vi "add_Control_panel.vi"(8 "error in (no error)":errorcluster, 10 "VI Refnum out":refnum<vi>, 11 "Control_Ref":refnum<vi>) -> (0 "error out":errorcluster, 3 "New Control Ref":refnum<vi>)   [LabVIEW 2015]
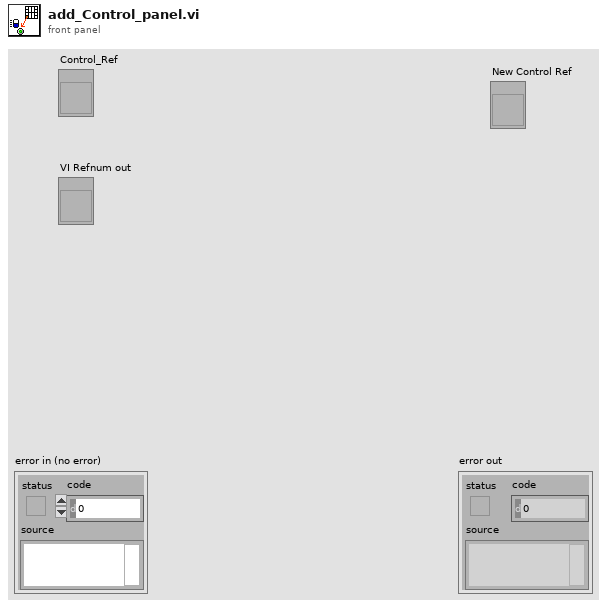
[diagram p1: front panel]
types:
  T1 = enum16{"Invalid Wire Rule", "Required", "Recommended", "Optional", "Dynamic Dispatch"}
  T2 = typedef "LVRectTypeDef.ctl" = cluster{"Left":i16, "Top":i16, "Right":i16, "Bottom":i16}
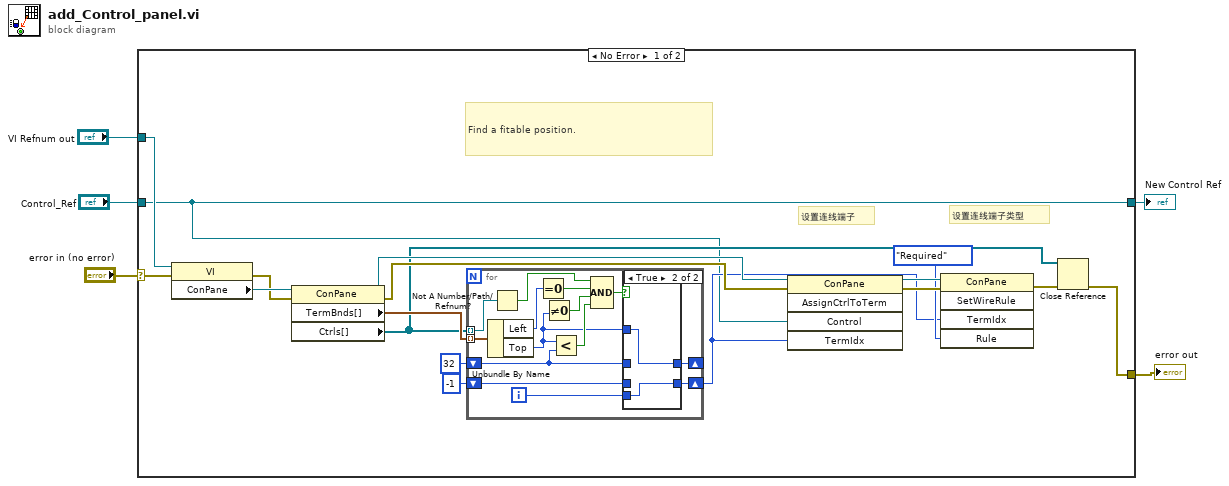
[diagram p0: block diagram]
diagram:
  n1 = case shown="No Error" "error in (no error)" {
    selector: "error in (no error)" -> [w8 w42]
    tunnel: [w7 w42] -> w4
    tunnel: "Control_Ref" -> [w6 w41]
    tunnel: "VI Refnum out" -> [w9 _]
    tunnel: [w6 w41] -> w1
    frame No Error {
      # "设置连线端子"
      # "设置连线端子类型"
      # "Find a fitable position."
      n2 = property class="VI"(reference=w9, error in=w8) -> (error out=w18:errorcluster, "ConPane"=w19:refnum<vi>)  [unwired: 1 out]
      n3 = property class="ConPane"(reference=w19, error in=w18) -> (reference out=w13:refnum<vi>, error out=w14:errorcluster, "TermBnds[]"=w15:T2[], "Ctrls[]"=w10:refnum<vi>[])
      n4 = for {
        tunnel: w15 -> [w26] mode=indexing
        shift-right: [w27] -> _
        shift-left: i16 32 -> [w31]
        shift-right: [w29] -> w12
        shift-left: -1 -> [w30]
        tunnel: w10 -> [w24] mode=indexing
        i -> [w28]
        n5 = Unbundle By Name(w26) -> ("Left"=w25:i16, "Top"=w32:i16)
        n6 = Not A Number/Path/Refnum?(number/path/refnum=w24) -> (NaN/Path/Refnum?=w23:bool)
        n7 = Equal To 0?(x=w25) -> (x = 0?=w36:bool)
        n8 = Not Equal To 0?(x=w32) -> (x != 0?=w35:bool)
        n9 = Less?(x=w32, y=w31) -> (x < y?=w34:bool)
        n10 = Compound Arithmetic op=AND(w23, w36, w35, w34) -> (w33:bool)
        n11 = case shown="True" w33 {
          tunnel: w32 -> [_ w39]
          tunnel: w31 -> [w38 _]
          tunnel: w30 -> [w37 _]
          tunnel: [w37 w40] -> w29
          tunnel: w28 -> [_ w40]
          tunnel: [w38 w39] -> w27
          frame False {
          }
          frame True {
          }
        }
      }
      n12 = invoke class="ConPane" method="AssignCtrlToTerm"(reference=w13, error in=w14, "Control"=w6, "TermIdx"=w12) -> (reference out=w21:refnum<vi>, error out=w22:errorcluster)  [unwired: 1 in, 3 out]
      n13 = invoke class="ConPane" method="SetWireRule"(reference=w21, error in=w22, "TermIdx"=w12, "Rule"=T1."Required") -> (error out=w11:errorcluster)  [unwired: 1 in, 4 out]
      n14 = Close Reference(reference=w10, error in (no error)=w11) -> (error out=w7:errorcluster)
    }
    frame Error {
    }
  }
  "error out" <- w4
  "New Control Ref" <- w1
